vi "rsmxo_LV2015_Trigger_Fetch_Waveform_Example.vi"() -> ()   [LabVIEW 2015]
uses:
  <instrlib>/Rohde&Schwarz MXO Oscilloscopes/Rohde&Schwarz MXO Oscilloscopes.lvlib
panel:
  in  "Record Length Limit":dbl=100000.0 caption="Record Length Limit (10000000)" format="%^.3e"
  in  "Time Scale":dbl=0.01 caption="Time Scale (20e-9)" format="%#.12p"
  in  "Coupling":i32(ring)=1 caption="Coupling (DC)" items=["DC", "DC Limit", "AC"]
  in  "Offset":dbl caption="Offset (0)" format="%#.12p"
  in  "Vertical Scale (per div)":dbl=0.1 caption="Vertical Scale (0.05)" format="%#.12p"
  out "Waveform Graph":T1(graph)={"X Start"=-0.05, "X Start"=1.0000000000000002e-08, "Waveform Data"=array[100000 elements]}
  in  "Trigger Level":dbl=0.05 caption="Level (0)" format="%#.12p"
  in  "Trigger Slope":i32(ring)=2 caption="Slope (Either)" items=["Positive", "Negative", "Either"]
  in  "Trigger Mode":i32(ring) caption="Trigger Mode (Auto)" items=["Auto", "Normal", "Free Run"]
  in  "Channel":i32(ring)=1 caption="Channel (1)" items=["1"=1, "2"=2, "3"=3, "4"=4, "External"=5]
  in  "VISA resource name":refnum<visa-resource-name>="TCPIP::10.205.0.159::hislip0"
  in  "Reset":bool
  in  "ID Query":bool=TRUE
  # "Rohde & Schwarz RTM2000 Oscilloscope Read Waveform Example"
  # "Rohde & Schwarz RTx Oscilloscopes Series\nTrigger-Fetch Waveform Example"
  # "Before running, change the VISA resource name to fit your device:\n- For LAN interface use TCPIP::<IP_Address>::INSTR e.g. TCPIP::10.64.0.178::INSTR\n- For USB interface use USB0::0x0AAD::<PID>::<SN>::INSTR e.g. USB0::0x0AAD::0x01D6::101457::INSTR\n- For GPIB interface use the GPIB::<Address>::INSTR e.g. GPIB::28::INSTR"
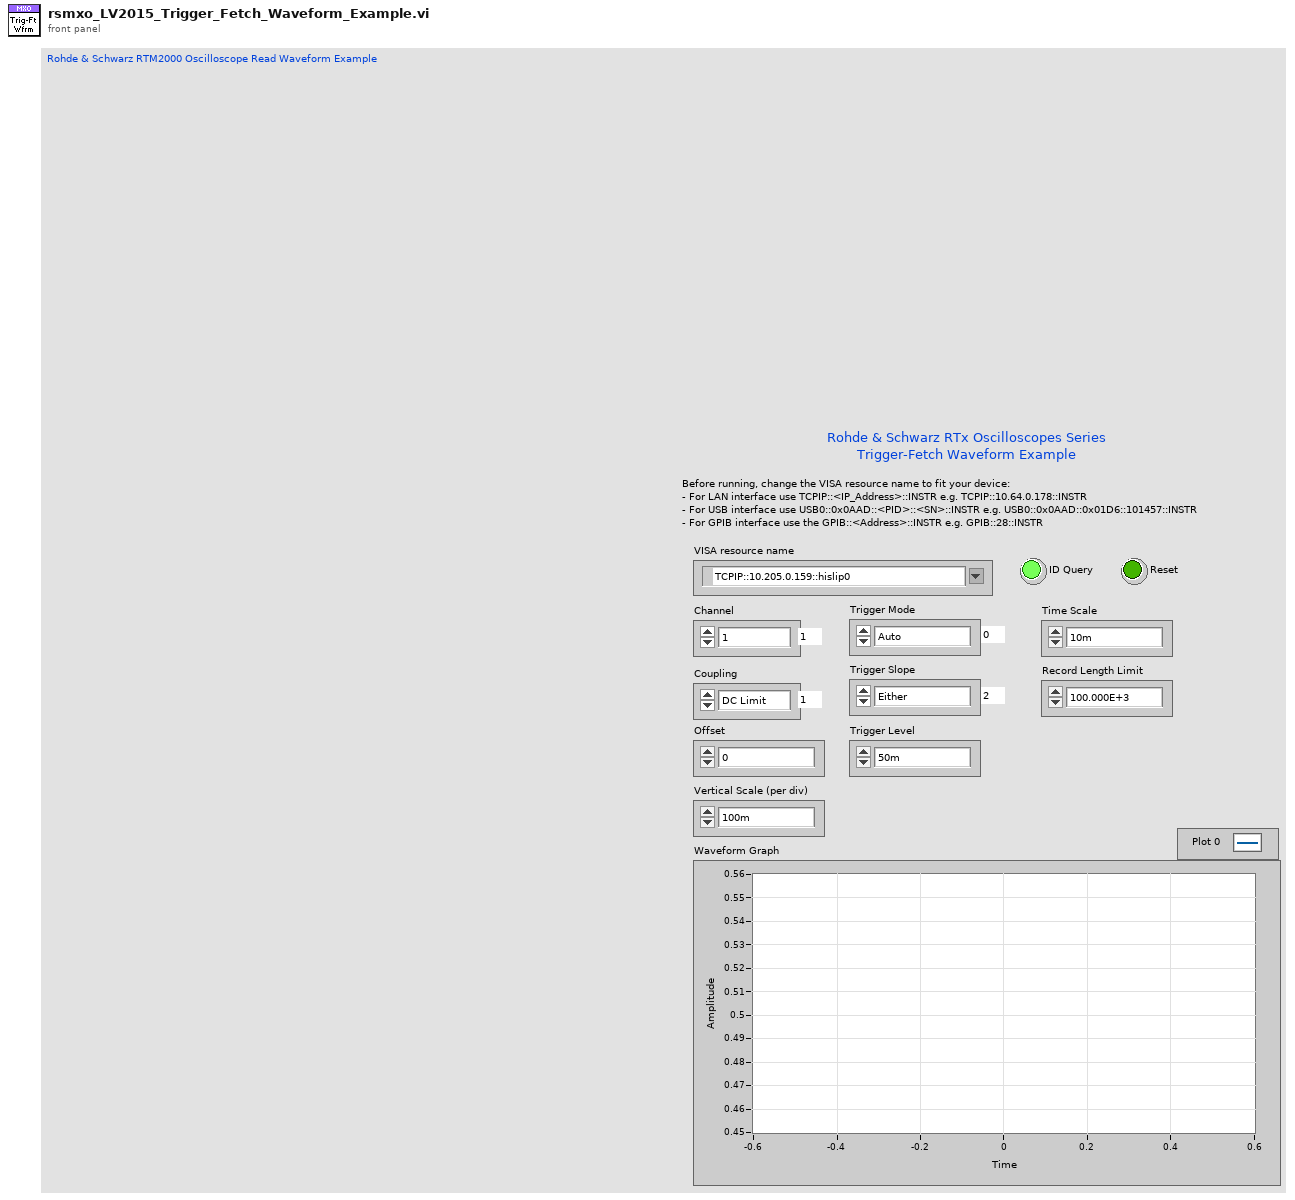
[diagram p1: front panel]
types:
  T1 = cluster{"X Start":dbl, "X Start":dbl, "Waveform Data":dbl[]}
  T2 = cluster{"X Start":dbl, dbl, "Waveform Data":dbl[]}
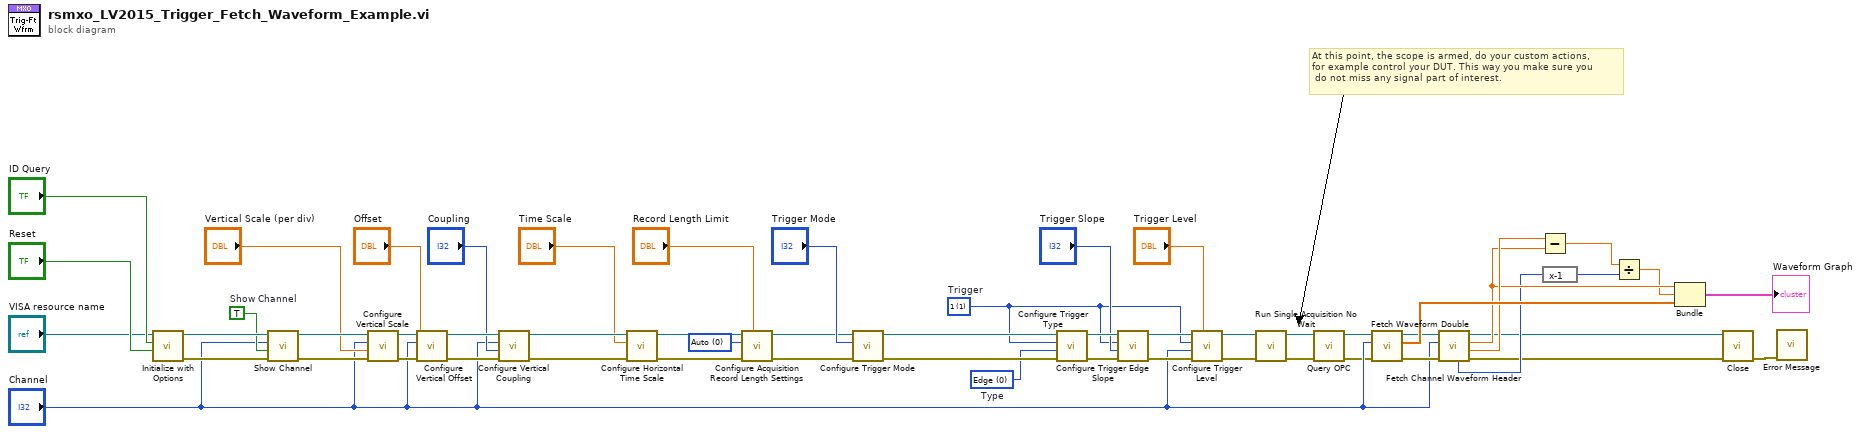
[diagram p0: block diagram]
diagram:
  w13 = 0 items=["Auto", "Manual"] ("Mode (Auto)")
  w24 = TRUE  # Show Channel
  w47 = 0 items=["Edge", "Glitch", "Width", "Runt", "Window", "Timeout", "Interval", "Slewrate", "Sethold", "State", "Pattern", "Analog Edge"]  # Type
  w41 = 1 items=["1"=1, "2"=2, "3"=3]  # Trigger
  # "At this point, the scope is armed, do your custom actions,\nfor example control your DUT. This way you make sure you\n do not miss any signal part of interest."
  n1 = call <instrlib>:"Initialize with Options.vi"("Reset (T: Reset)"="Reset", "ID Query (T: Check)"="ID Query", "VISA resource name"="VISA resource name") -> ("error out"=w32:errorcluster, "VISA resource name out"=w31:refnum<visa-resource-name>)  [unwired: 7 in]
  n2 = call <instrlib>:"Show Channel.vi"("error in (no error)"=w32, "Show Channel (Off)"=w24, "Channel (1)"="Channel", "VISA resource name"=w31) -> ("error out"=w30:errorcluster, "VISA resource name out"=w29:refnum<visa-resource-name>)  [unwired: 6 in]
  n3 = call <instrlib>:"Configure Vertical Scale.vi"("error in (no error)"=w30, "Vertical Scale (0.05)"="Vertical Scale (per div)", "Channel (1)"="Channel", "VISA resource name"=w29) -> ("error out"=w28:errorcluster, "VISA resource name out"=w27:refnum<visa-resource-name>)  [unwired: 6 in]
  n4 = call <instrlib>:"Configure Vertical Offset.vi"("error in (no error)"=w28, "Offset (0)"="Offset", "Channel (1)"="Channel", "VISA resource name"=w27) -> ("error out"=w26:errorcluster, "VISA resource name out"=w25:refnum<visa-resource-name>)  [unwired: 6 in]
  n5 = call <instrlib>:"Configure Vertical Coupling.vi"("error in (no error)"=w26, "Coupling (DC)"="Coupling", "Channel (1)"="Channel", "VISA resource name"=w25) -> ("error out"=w20:errorcluster, "VISA resource name out"=w19:refnum<visa-resource-name>)  [unwired: 6 in]
  n6 = call <instrlib>:"Configure Horizontal Time Scale.vi"("error in (no error)"=w20, "Time Scale (20e-9)"="Time Scale", "VISA resource name"=w19) -> ("error out"=w17:errorcluster, "VISA resource name out"=w16:refnum<visa-resource-name>)  [unwired: 7 in]
  n7 = call <instrlib>:"Configure Acquisition Record Length Settings.vi"("Record Length Limit (10000000)"="Record Length Limit", "error in (no error)"=w17, "Mode (Auto)"=w13, "VISA resource name"=w16) -> ("error out"=w15:errorcluster, "VISA resource name out"=w14:refnum<visa-resource-name>)  [unwired: 6 in]
  n8 = call <instrlib>:"Configure Trigger Mode.vi"("error in (no error)"=w15, "Trigger Mode (Auto)"="Trigger Mode", "VISA resource name"=w14) -> ("error out"=w50:errorcluster, "VISA resource name out"=w49:refnum<visa-resource-name>)  [unwired: 7 in]
  n9 = call <instrlib>:"Configure Trigger Type.vi"("error in (no error)"=w50, "Type (Edge)"=w47, "Trigger (1)"=w41, "VISA resource name"=w49) -> ("error out"=w46:errorcluster, "VISA resource name out"=w45:refnum<visa-resource-name>)  [unwired: 6 in]
  n10 = call <instrlib>:"Configure Trigger Edge Slope.vi"("error in (no error)"=w46, "Slope (Either)"="Trigger Slope", "Trigger (1)"=w41, "VISA resource name"=w45) -> ("error out"=w44:errorcluster, "VISA resource name out"=w43:refnum<visa-resource-name>)  [unwired: 6 in]
  n11 = call <instrlib>:"Configure Trigger Level.vi"("Level (0)"="Trigger Level", "error in (no error)"=w44, "Channel (1)"="Channel", "Trigger (1)"=w41, "VISA resource name"=w43) -> ("error out"=w6:errorcluster, "VISA resource name out"=w5:refnum<visa-resource-name>)  [unwired: 5 in]
  n12 = call <instrlib>:"Run Single Acquisition No Wait.vi"("error in (no error)"=w6, "VISA resource name"=w5) -> ("error out"=w4:errorcluster, "VISA resource name out"=w3:refnum<visa-resource-name>)  [unwired: 8 in]
  n13 = call <instrlib>:"Query OPC.vi"("error in (no error)"=w4, "VISA resource name"=w3) -> ("error out"=w2:errorcluster, "VISA resource name out"=w1:refnum<visa-resource-name>)  [unwired: 7 in, 1 out]
  n14 = call <instrlib>:"Fetch Waveform Double.vi"("error in (no error)"=w2, "Source (Channel 1)"="Channel", "VISA resource name"=w1) -> ("error out"=w11:errorcluster, "Waveform Data"=w52:dbl[], "VISA resource name out"=w10:refnum<visa-resource-name>)  [unwired: 6 in]
  n15 = call <instrlib>:"Fetch Channel Waveform Header.vi"("error in (no error)"=w11, "Channel (1)"="Channel", "VISA resource name"=w10) -> ("error out"=w8:errorcluster, "X Stop"=w38:dbl, "X Start"=w37:dbl, "VISA resource name out"=w7:refnum<visa-resource-name>, "Record Length"=w35:i32)  [unwired: 3 in, 1 out]
  n16 = Subtract(x=w38, y=w37) -> (x-y=w36:dbl)
  n17 = expression code="x-1"(w35) -> (w34:i32)
  n18 = Divide(x=w36, y=w34) -> (x/y=w33:dbl)
  n19 = Bundle("X Start"=w37, w33, "Waveform Data"=w52) -> (→"Waveform Graph":T2)  [unwired: 1 in]
  n20 = call <instrlib>:"Close.vi"("error in (no error)"=w8, "VISA resource name"=w7) -> ("error out"=w51:errorcluster)  [unwired: 9 in]
  n21 = call <instrlib>:"Error Message.vi"("error in (no error)"=w51) -> ()  [unwired: 10 in, 5 out]
